vi "galvoGeneratePositionsGrid.vi"(1 "N-1":i32) -> (0 "grid":dbl[][](array[numeric]))   [LabVIEW 2017]
uses:
  globalDevices.vi
panel:
  # "Returns a 2D grid in fractional units [-1,+1]\nas a 1D array of [X,Y]."
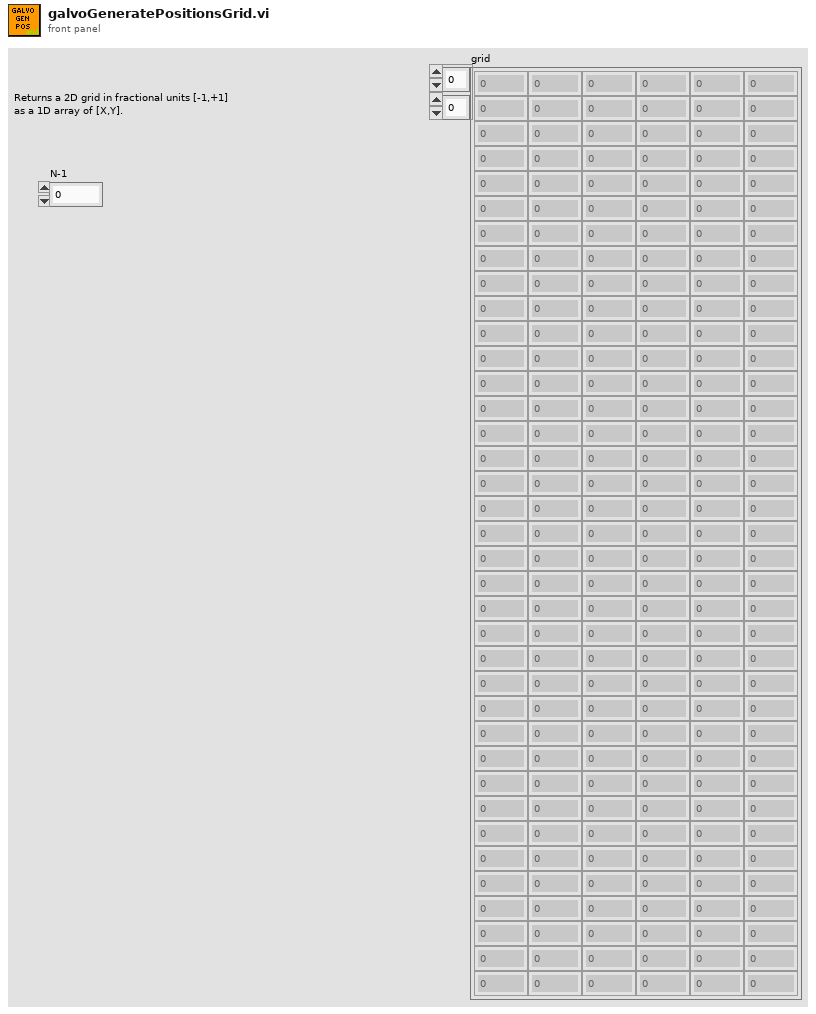
[diagram p1: front panel]
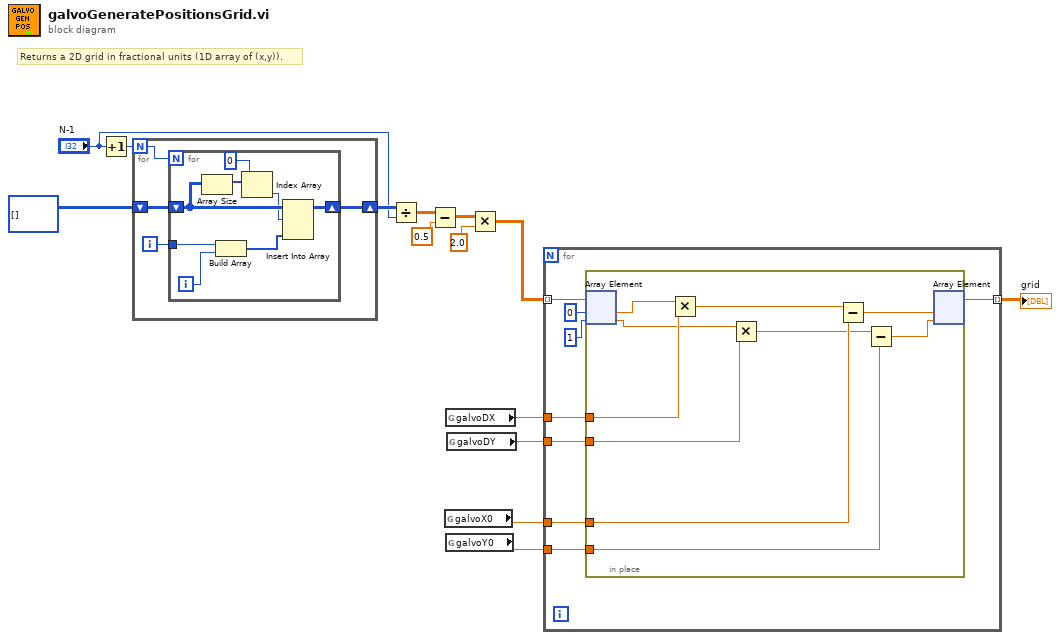
[diagram p0: block diagram]
diagram:
  # "Returns a 2D grid in fractional units (1D array of (x,y))."
  n1 = Increment(x="N-1") -> (x+1=w7:i32)
  n2 = for {
    N: w7 -> [w15]
    shift-right: [w16] -> w13
    shift-left: i32[][] [] -> [w17]
    i -> [w18]
    n3 = for {
      N: w15 -> [_]
      tunnel: w18 -> [w25]
      shift-right: [w24] -> w16
      shift-left: w17 -> [w21]
      i -> [w26]
      n4 = Array Size(array=w21) -> (size(s)=w23:i32[])
      n5 = Build Array(w25, w26) -> (w19:i32[])
      n6 = Index Array(array=w23, index=0) -> (element=w20:i32)
      n7 = Insert Into Array(array=w21, index (row)=w20, new element=w19) -> (w24:i32[][])  [unwired: 1 in]
    }
  }
  n8 = Divide(x=w13, y="N-1") -> (x/y=w11:dbl[][])
  n9 = Subtract(x=w11, y=0.5) -> (x-y=w9:dbl[][])
  n10 = global read "globalDevices.vi" "galvoX0"() -> (w5:dbl)
  n11 = global read "globalDevices.vi" "galvoDX"() -> (w1:dbl)
  n12 = global read "globalDevices.vi" "galvoY0"() -> (w4:dbl)
  n13 = global read "globalDevices.vi" "galvoDY"() -> (w2:dbl)
  n14 = Multiply(x=w9, y=2.0) -> (x*y=w6:dbl[][])
  n15 = for {
    tunnel: w6 -> [w34] mode=indexing
    tunnel: w5 -> [w31]
    tunnel: w4 -> [w30]
    tunnel: [w29] -> w3 mode=indexing
    tunnel: w2 -> [w28]
    tunnel: w1 -> [w27]
    n16 = in-place {
      in-place-border: w31 -> [w44]
      in-place-border: w30 -> [w42]
      in-place-border: w28 -> [w37]
      in-place-border: w27 -> [w39]
      n17 = in-place-array #1(w34, 0, 1) -> (w40:dbl, w38:dbl)
      n18 = Multiply(x=w40, y=w39) -> (x*y=w36:dbl)
      n19 = Multiply(x=w38, y=w37) -> (x*y=w35:dbl)
      n20 = Subtract(x=w36, y=w44) -> (x-y=w43:dbl)
      n21 = Subtract(x=w35, y=w42) -> (x-y=w41:dbl)
      n22 = in-place-array #1(w43, w41) -> (w29:dbl[])  [unwired: 2 out]
    }
  }
  "grid" <- w3
